vi "Mode Shift Action.vi"(7 "Error In":errorcluster, 8 "MS Requested State":T2, 9 "GEA Inputs":T1 {"Destination" format="%.0x"; "Source" format="%.0x"}, 10 "Standalone?":bool, 11 "GEA2 Reference In":refnum<k24>) -> (0 "Error Out":errorcluster, 2 "MS State":string, 3 "GEA2 Reference Out":refnum<k24>)   [LabVIEW 2016, in "TL27.lvlib"]
uses:
  Projects/TL27.lvlib
  type defs/Mode Shift Requested State.ctl
  C:/Automation/DLLs/PC Dot Net/GeaCommunication.dll
  Common/LabVIEW GEA2 Toolkit/LabVIEW_GEA2_Toolkit.lvlibp/type defs/Source_Destination.ctl
  Common/LabVIEW GEA2 Toolkit/LabVIEW_GEA2_Toolkit.lvlibp/type defs/ERD Read Data In.ctl
  Common/LabVIEW GEA2 Toolkit/LabVIEW_GEA2_Toolkit.lvlibp/type defs/Data Type.ctl
  Common/LabVIEW GEA2 Toolkit/LabVIEW_GEA2_Toolkit.lvlibp/type defs/ERD Write Data In.ctl
  Common/LabVIEW GEA2 Toolkit/LabVIEW_GEA2_Toolkit.lvlibp
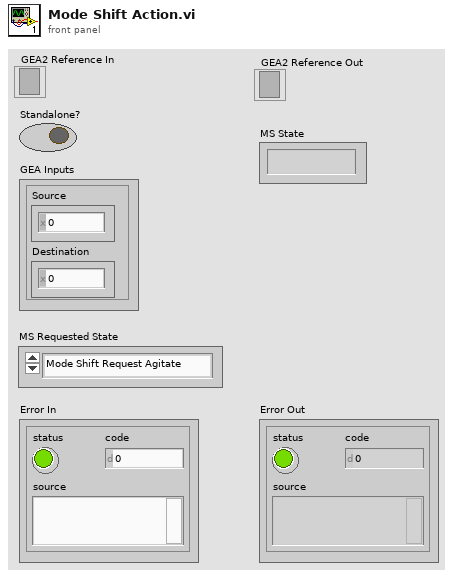
[diagram p1: front panel]
types:
  T1 = typedef "LabVIEW_GEA2_Toolkit.lvlibp/Source_Destination.ctl" = cluster{"Source":u8, "Destination":u8}
  T2 = typedef "TL27.lvlib/Mode Shift Requested State.ctl" = enum16{"Mode Shift Request Agitate", "Mode Shift Request Spin"}
  T3 = typedef "LabVIEW_GEA2_Toolkit.lvlibp/ERD Read Data In.ctl" = cluster{"ERD Number":u16, "Data Type":T4}
  T4 = typedef "LabVIEW_GEA2_Toolkit.lvlibp/Data Type.ctl" = enum16{"string", "boolean", "uint8_t", "uint16_t", "uint32_t", "uint64_t", "int8_t", "int16_t", "int32_t", "int64_t"}
  T5 = typedef "LabVIEW_GEA2_Toolkit.lvlibp/ERD Read Data Out.ctl" = cluster{"ERD Number":u16, "Data":string}
  T6 = typedef "LabVIEW_GEA2_Toolkit.lvlibp/ERD Write Data In.ctl" = cluster{"ERD Number":u16, "Data Type":T4, "Data":string}
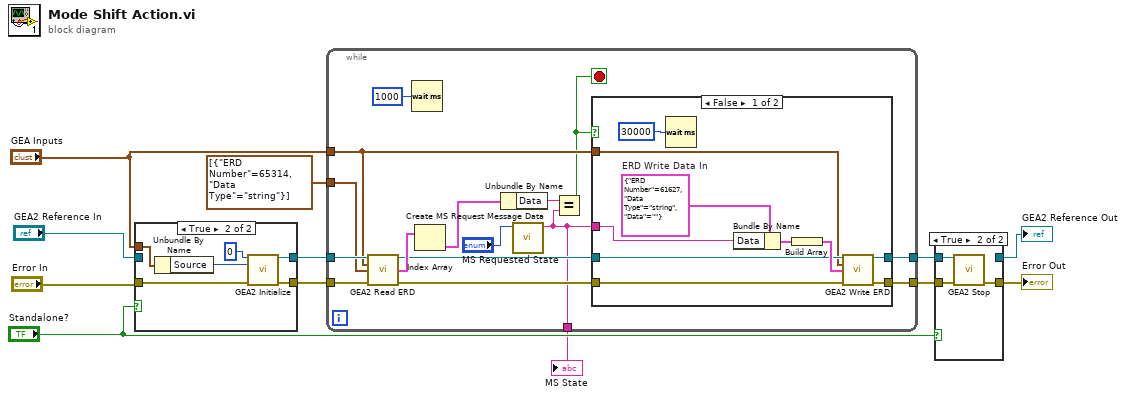
[diagram p0: block diagram]
diagram:
  n1 = case shown="True" "Standalone?" {
    tunnel: "Error In" -> [w13 w20]
    tunnel: [w13 w19] -> w12
    tunnel: "GEA2 Reference In" -> [w14 _]
    tunnel: [w14 w18] -> w7
    tunnel: "GEA Inputs" -> [_ w16]
    frame False {
    }
    frame True {
      n2 = Unbundle By Name(w16) -> ("Source"=w17:u8)
      n3 = call "GEA2 Initialize.vi"("Board Index"=0, "Source Address"=w17, "error in"=w20) -> ("GEA2 Reference Out"=w18:refnum<k24>, "error out"=w19:errorcluster)  [unwired: 10 in, 1 out]
    }
  }
  n4 = while {
    tunnel: w12 -> [w34]
    tunnel: w7 -> [w30]
    tunnel: [w29] -> w6
    tunnel: [w27] -> w5
    tunnel: T3[] [{"ERD Number"=65314, "Data Type"=enum."string"}] ("Read ERD List") -> [w25]
    tunnel: "GEA Inputs" -> [w24]
    tunnel: [w22] -> w1
    stop <- w23 stop-if-true
    n5 = call "GEA2 Read ERD.vi"("GEA2 Reference In"=w30, "GEA Inputs"=w24, "Read ERD List"=w25, "Error In"=w34) -> ("GEA2 Reference Out"=w28:refnum<k24>, "ERD Data Out"=w33:T5[], "Error Out"=w26:errorcluster)  [unwired: 8 in, 1 out]
    n6 = Wait (ms)(milliseconds to wait=u32 1000) -> ()  [unwired: 1 out]
    n7 = Index Array(array=w33) -> (element=w32:T5)  [unwired: 1 in]
    n8 = Unbundle By Name(w32) -> ("Data"=w31:string)
    n9 = call "Create MS Request Message Data .vi"("MS Requested State"="MS Requested State") -> ("MS State"=w22:string)  [unwired: 10 in]
    n10 = Equal?(x=w31, y=w22) -> (x = y?=w23:bool)
    n11 = case shown="False" w23 {
      tunnel: w26 -> [w42 w46]
      tunnel: [w41 w46] -> w29
      tunnel: w28 -> [w40 w47]
      tunnel: [w37 w47] -> w27
      tunnel: w22 -> [w39 _]
      tunnel: w24 -> [w38 _]
      frame False {
        w45 = T6 {"ERD Number"=61627, "Data Type"=enum."string", "Data"=""}  # ERD Write Data In
        n12 = Wait (ms)(milliseconds to wait=u32 30000) -> ()  [unwired: 1 out]
        n13 = Bundle By Name(cluster=w45, "Data"=w39) -> (w44:T6)
        n14 = Build Array(w44) -> (w43:T6[])
        n15 = call "GEA2 Write ERD.vi"("GEA2 Reference In"=w40, "GEA Inputs"=w38, "Write ERD List"=w43, "Error In"=w42) -> ("GEA2 Reference Out"=w37:refnum<k24>, "Error Out"=w41:errorcluster)  [unwired: 9 in, 1 out]
      }
      frame True {
      }
    }
  }
  "MS State" <- w1
  n16 = case shown="True" "Standalone?" {
    tunnel: w6 -> [w48 w52]
    tunnel: [w48 w51] -> w10
    tunnel: w5 -> [w49 w50]
    tunnel: [w49 _] -> w8
    frame False {
    }
    frame True {
      n17 = call "GEA2 Stop.vi"("GEA2 Reference In"=w50, "Error In"=w52) -> ("Error Out"=w51:errorcluster)  [unwired: 13 in]
    }
  }
  "Error Out" <- w10
  "GEA2 Reference Out" <- w8
